vi "CalcIncr.vi"(8 "error in (no error)":errorcluster, 10 "Curr Iter Params":T1, 11 "PosCtrl Params":T2) -> (0 "error out":errorcluster, 2 "Bow Reference":dbl, 3 "Incremental step":dbl, 5 "Step Completed?":bool)   [LabVIEW 2020, in "PlannedMotionSequence.lvlib"]
doc: "Calculate incremental step size with sign based on direction for the next iteration. Also check if this step is completed. (PosCtrl mode)"
uses:
  PlannedMotionSequence.lvlib
  TypeDefs/PosCtrl Params.ctl
  TypeDefs/CurrIterParams.ctl
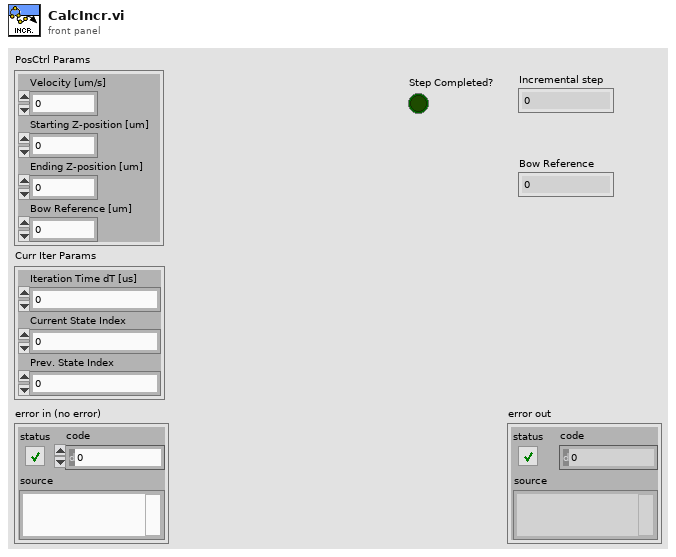
[diagram p1: front panel]
types:
  T1 = typedef "PlannedMotionSequence.lvlib/CurrIterParams.ctl" = cluster{"Iteration Time dT [us]":dbl, "Current State Index":i32, "Prev. State Index":i32}
  T2 = typedef "PlannedMotionSequence.lvlib/PosCtrl Params.ctl" = cluster{"Velocity [um/s]":dbl, "Starting Z-position [um]":dbl, "Ending Z-position [um]":dbl, "Bow Reference [um]":dbl}
  T3 = cluster{dbl, "Ending Z-position [um]":dbl, "Bow Reference [um]":dbl}
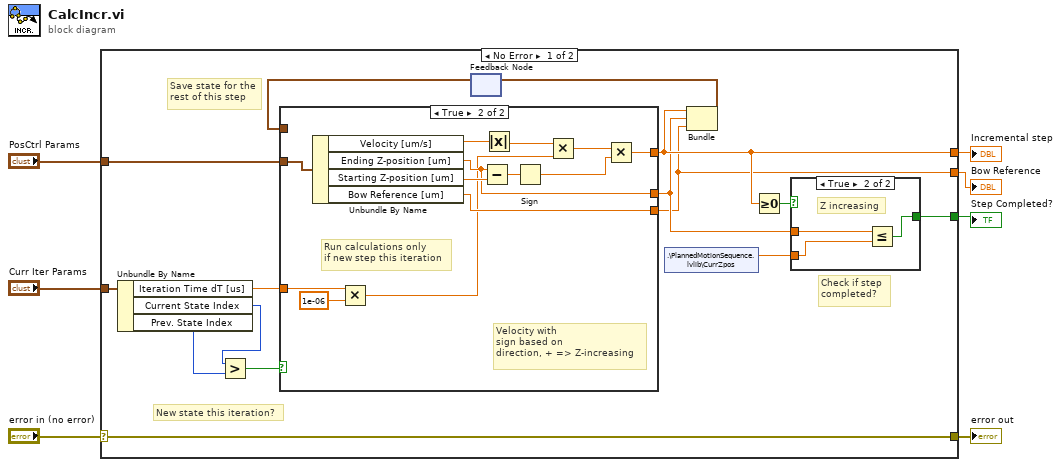
[diagram p0: block diagram]
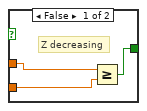
[diagram p2: hidden frame]
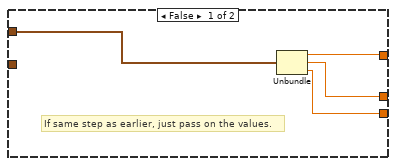
[diagram p3: hidden frame]
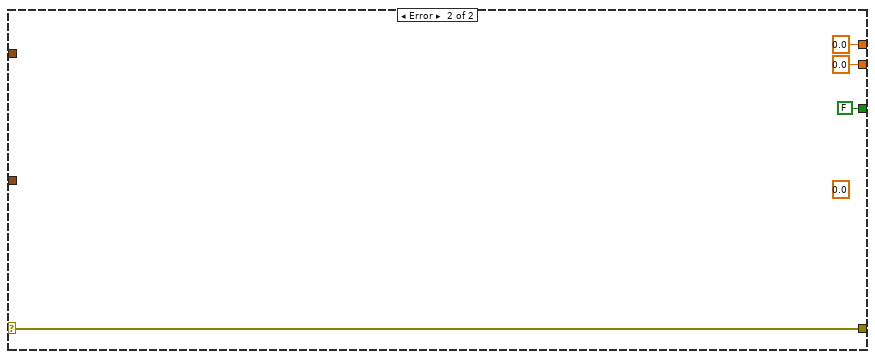
[diagram p4: hidden frame]
diagram:
  n1 = case shown="No Error" "error in (no error)" {
    selector: "error in (no error)" -> [w15 w49]
    tunnel: [w15 w49] -> w6
    tunnel: "Curr Iter Params" -> [w22 _]
    tunnel: "PosCtrl Params" -> [w20 _]
    tunnel: [w13 0.0] -> w3
    tunnel: [w11 FALSE] -> w2
    tunnel: [w9 0.0 ("Bow Reference [um]")] -> w1
    frame No Error {
      # "Check if step\ncompleted?"
      # "Save state for the\nrest of this step"
      # "New state this iteration?"
      n2 = Unbundle By Name(w22) -> ("Iteration Time dT [us]"=w19:dbl, "Current State Index"=w21:i32, "Prev. State Index"=w8:i32)
      n3 = Greater?(x=w21, y=w8) -> (0:w18:bool)
      n4 = feedback #1() -> (w16:T3)  [unwired: 1 in]
      n5 = case shown="True" w18 {
        tunnel: w20 -> [_ w45]
        tunnel: w19 -> [_ w35]
        tunnel: [w31 w39] -> w13
        tunnel: w16 -> [w32 _]
        tunnel: [w30 w37] -> w12
        tunnel: [w29 w36] -> w9
        frame False {
          # "If same step as earlier, just pass on the values."
          n6 = Unbundle(w32) -> (w31:dbl, "Ending Z-position [um]"=w30:dbl, "Bow Reference [um]"=w29:dbl)
        }
        frame True {
          # "Run calculations only \nif new step this iteration"
          # "Velocity with \nsign based on \ndirection, + => Z-increasing"
          n7 = Unbundle By Name(w45) -> ("Velocity [um/s]"=w44:dbl, "Ending Z-position [um]"=w37:dbl, "Starting Z-position [um]"=w41:dbl, "Bow Reference [um]"=w36:dbl)
          n8 = Multiply(x=w35, y=1e-06) -> (x*y=w33:dbl)
          n9 = Subtract(x=w37, y=w41) -> (x-y=w40:dbl)
          n10 = Absolute Value(x=w44) -> (abs(x)=w42:dbl)
          n11 = Sign(1:w40) -> (0:w38:dbl)
          n12 = Multiply(x=w42, y=w33) -> (x*y=w43:dbl)
          n13 = Multiply(x=w43, y=w38) -> (x*y=w39:dbl)
        }
      }
      n14 = shared-variable ".\\PlannedMotionSequence.lvlib\\CurrZpos"() -> (w10:dbl)  [unwired: 1 in, 1 out]
      n15 = Bundle(w13, "Ending Z-position [um]"=w12, "Bow Reference [um]"=w9) -> (w17:T3)  [unwired: 1 in]
      n16 = feedback-in #1(w17) -> ()
      n17 = Greater Or Equal To 0?(x=w13) -> (x >= 0?=w14:bool)
      n18 = case shown="True" w14 {
        tunnel: [w25 w28] -> w11
        tunnel: w10 -> [w24 w27]
        tunnel: w12 -> [w23 w26]
        frame False {
          # "Z decreasing"
          n19 = Greater Or Equal?(x=w23, y=w24) -> (x >= y?=w25:bool)
        }
        frame True {
          # "Z increasing"
          n20 = Less Or Equal?(x=w26, y=w27) -> (x <= y?=w28:bool)
        }
      }
    }
    frame Error {
      (unwired) 0.0 ("Double")
    }
  }
  "error out" <- w6
  "Incremental step" <- w3
  "Step Completed?" <- w2
  "Bow Reference" <- w1
